vi "test_speckle_mask.vi"() -> ()   [LabVIEW 2016]
uses:
  <vilib>/vision/NI_Vision_Development_Module.lvlib
panel:
  out "0, 1":i16[][](array[numeric])
  out "Boolean Mask":i16[][](graph)
  out "Image":T1(plugin-control)
  out "Mask (Image)":T1(plugin-control)
  in  "Threshold Multiplier":sgl=2.0
  out "Counter":i32
  out "Num Images":dbl=1000.0
  in  "AVI File for Simulated Raw B Scan Images":path=path "C:/Users/Applied Optics Group/Desktop/DCF Paper Data Processing/data/2020_08_04_2dcheckerboard_AF/Large_grid/OCT_raw_vol.avi"
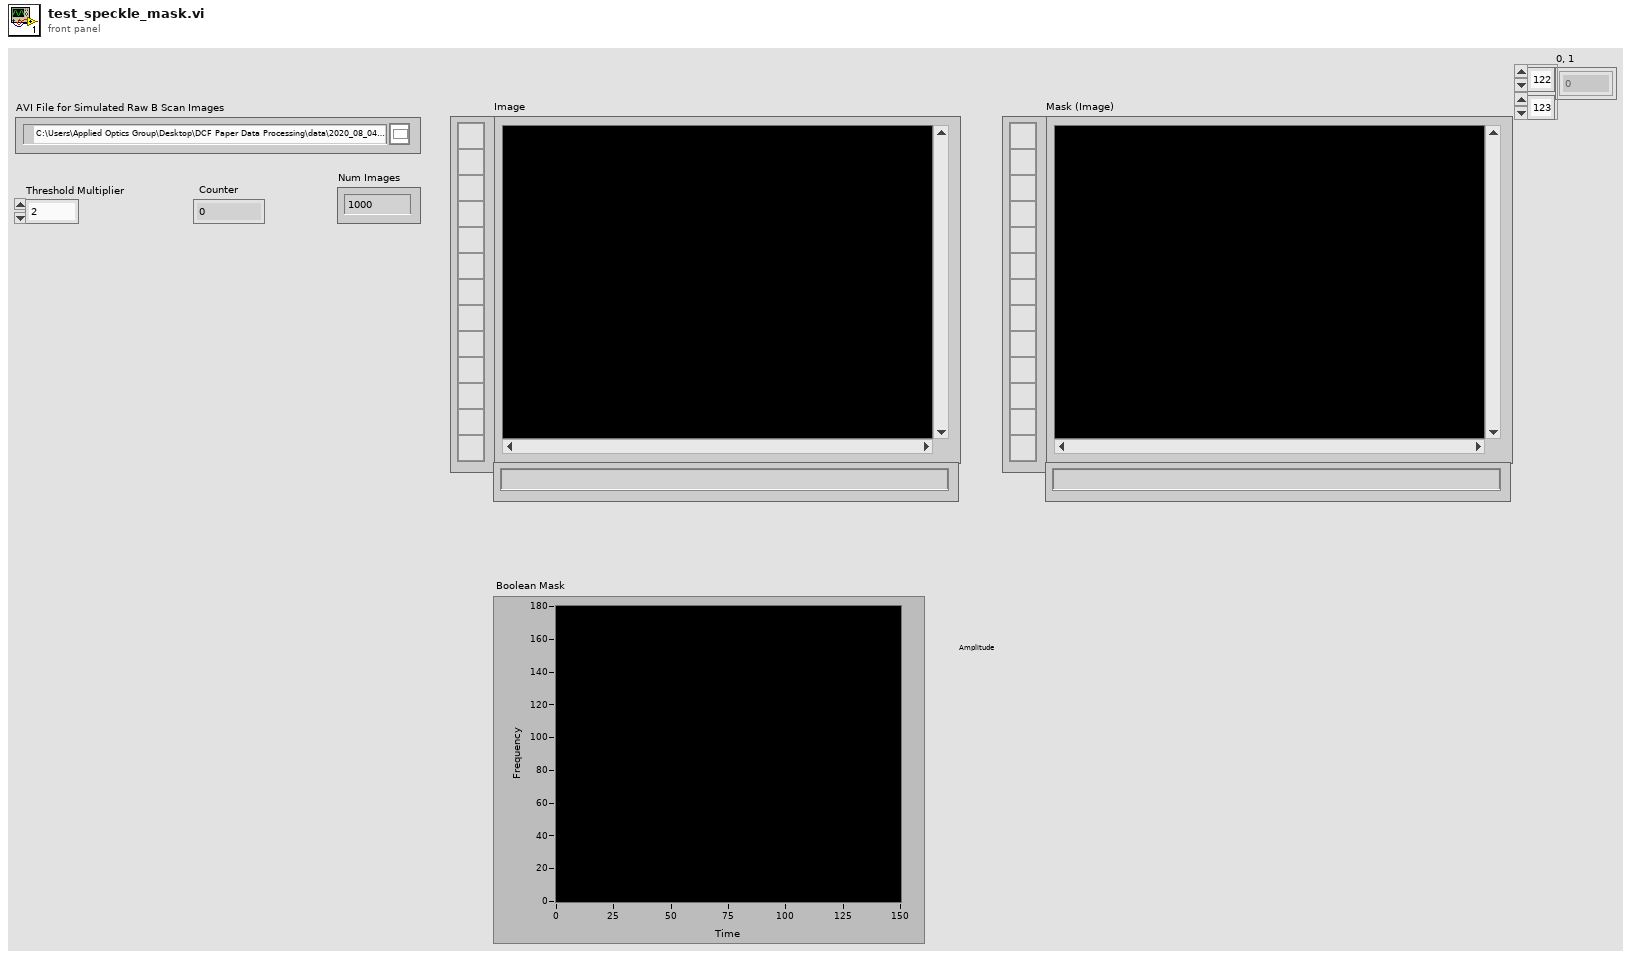
[diagram p1: front panel]
types:
  T1 = typedef "IMAQ Image.ctl" = refnum<image>
  T2 = typedef "Image Type" = u32
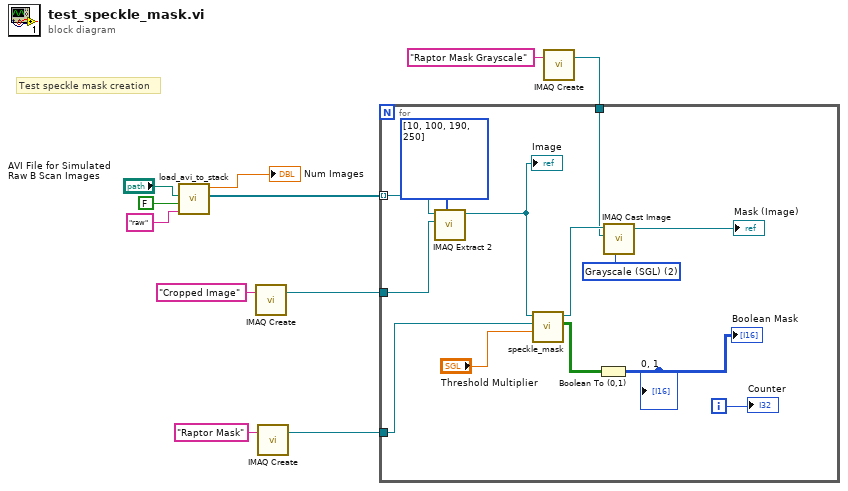
[diagram p0: block diagram]
diagram:
  # "Test speckle mask creation"
  n1 = call "load_avi_to_stack.vi"("Image Prefix"="raw", "Preview"=FALSE, "AVI File"="AVI File for Simulated Raw B Scan Images") -> ("Image Array"=w7:T1[], "Num Images"=→"Num Images":dbl)  [unwired: 7 in]
  n2 = call "IMAQ Create"("Image Name"="Cropped Image") -> ("New Image"=w3:T1)  [unwired: 4 in, 1 out]
  n3 = call "IMAQ Create"("Image Name"="Raptor Mask") -> ("New Image"=w5:T1)  [unwired: 4 in, 1 out]
  n4 = call "IMAQ Create"("Image Name"="Raptor Mask Grayscale") -> ("New Image"=w1:T1)  [unwired: 4 in, 1 out]
  n5 = for {
    tunnel: w7 -> [w20] mode=indexing
    tunnel: w5 -> [w23]
    tunnel: w3 -> [w21]
    tunnel: w1 -> [w14]
    i -> [w24]
    w15 = T2 2 items=["Grayscale (U8)", "Grayscale (I16)", "Grayscale (SGL)", "Complex (CSG)", "RGB (U32)", "HSL (U32)", "RGB (U64)", "Grayscale (U16)"] ("Image Type")
    n6 = call "IMAQ Extract 2"("Optional Rectangle"=i32[] [10, 100, 190, 250], "Image Dst"=w21, "Image Src"=w20) -> ("Image Dst Out"=w18:T1)  [unwired: 7 in, 1 out]
    "Image" <- w18
    n7 = call "speckle_mask.vi"("Threshold Multiplier"="Threshold Multiplier", "Image Out"=w23, "Image In"=w18) -> ("Mask Out"=w13:bool[][], "Image Dst Out"=w16:T1)  [unwired: 6 in, 1 out]
    n8 = Boolean To (0,1)(Boolean=w13) -> (0, 1=→"Boolean Mask" →"0, 1":i16[][])
    n9 = call "IMAQ Cast Image"("Image Type"=w15, "Image Dst"=w14, "Image Src"=w16) -> ("Image Dst Out"=→"Mask (Image)":T1)  [unwired: 7 in, 1 out]
    "Counter" <- w24
  }
